vi "Add Available Device.vi"(8 "error in (no error)":errorcluster, 9 "Type":string, 10 "Device":refnum<class "Device.lvclass">, 11 "HAL Editor in":refnum<class "HAL Editor.lvclass">) -> (0 "error out":errorcluster, 3 "HAL Editor out":refnum<class "HAL Editor.lvclass">)   [LabVIEW 2012, in "HAL Config.lvlib" / "HAL Editor.lvclass"]
uses:
  HAL Editor.lvclass
  build/ppl/lv-hal.lvlibp/Device/Device.lvclass
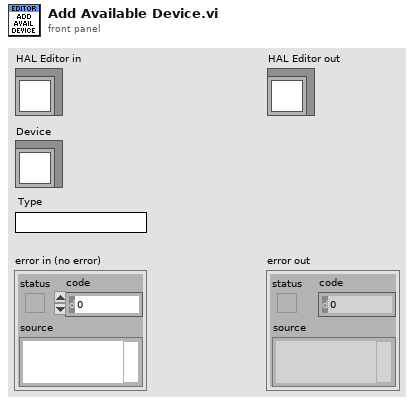
[diagram p1: front panel]
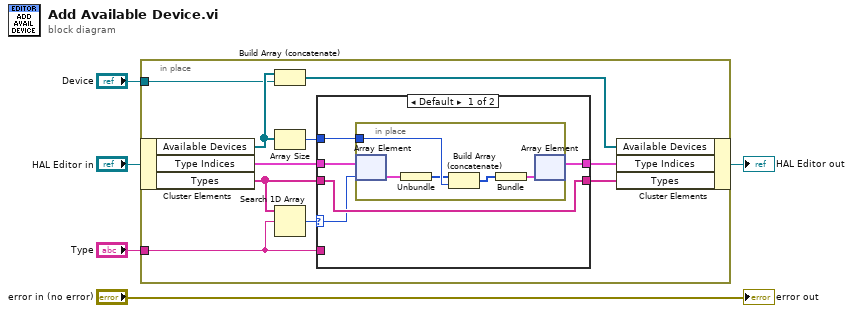
[diagram p0: block diagram]
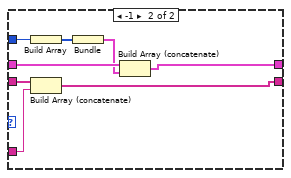
[diagram p2: hidden frame]
diagram:
  n1 = in-place {
    in-place-border: "Type" -> [w8]
    in-place-border: "Device" -> [w11]
    n2 = in-place-cluster #1("HAL Editor in") -> ("Available Devices"=w12:refnum<class "Device.lvclass">[], "Type Indices"=w13:cluster{"Indices":i32[]}[], "Types"=w14:string[])
    n3 = Build Array (concatenate)(w12, w11) -> (w9:refnum<class "Device.lvclass">[])
    n4 = Array Size(array=w12) -> (size(s)=w10:i32)
    n5 = Search 1D Array(1D array=w14, element=w8) -> (index of element=w15:i32)  [unwired: 1 in]
    n6 = case shown="Default" w15 {
      selector: w15 -> [w18 _]
      tunnel: w14 -> [w20 w33]
      tunnel: w13 -> [w19 w29]
      tunnel: w10 -> [w17 w31]
      tunnel: w8 -> [_ w32]
      tunnel: [w20 w26] -> w7
      tunnel: [w16 w27] -> w6
      frame Default {
        n7 = in-place {
          in-place-border: w17 -> [w24]
          n8 = in-place-array #2(w19, w18) -> (w25:cluster{"Indices":i32[]})
          n9 = Unbundle(w25) -> ("Indices"=w23:i32[])
          n10 = Build Array (concatenate)(w23, w24) -> (w22:i32[])
          n11 = Bundle(w22) -> (w21:cluster{i32[]})  [unwired: 1 in]
          n12 = in-place-array #2(w21) -> (w16:cluster{"Indices":i32[]}[])  [unwired: 1 out]
        }
      }
      frame -1 {
        n13 = Build Array(w31) -> (w30:i32[])
        n14 = Build Array (concatenate)(w33, w32) -> (w26:string[])
        n15 = Bundle(w30) -> (w28:cluster{i32[]})  [unwired: 1 in]
        n16 = Build Array (concatenate)(w29, w28) -> (w27:cluster{"Indices":i32[]}[])
      }
    }
    n17 = in-place-cluster #1("Available Devices"=w9, "Type Indices"=w6, "Types"=w7) -> (→"HAL Editor out":refnum<class "HAL Editor.lvclass">)
  }
  "error out" <- "error in (no error)"
